vi "Que values for sending.vi"() -> (0 "error out":errorcluster, 1 "queue out":refnum<queue>)   [LabVIEW 2016]
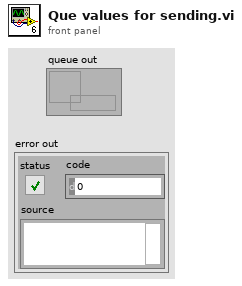
[diagram p1: front panel]
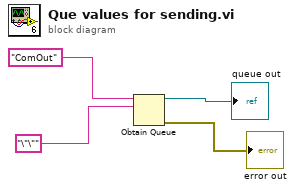
[diagram p0: block diagram]
diagram:
  n1 = Obtain Queue(name (unnamed)="ComOut", element data type="\"\"" ("name (unnamed)")) -> (queue out=→"queue out":refnum<queue>, error out=→"error out":errorcluster)  [unwired: 3 in, 1 out]
